vi "Lookup API by ID.vi"(8 "error in (no error)":errorcluster, 10 "API ID":string, 11 "VolatusCoreTask in":refnum<class "VolatusCoreTask.lvclass">) -> (0 "error out":errorcluster, 2 "API":refnum<class "API.lvclass">, 3 "VolatusCoreTask out":refnum<class "VolatusCoreTask.lvclass">)   [LabVIEW 2020, in "Volatus.lvlib" / "VolatusCoreTask.lvclass"]
uses:
  VolatusCoreTask.lvclass
  VolatusCoreTask.lvclass/VolatusCoreTask.ctl
  API/API.lvclass
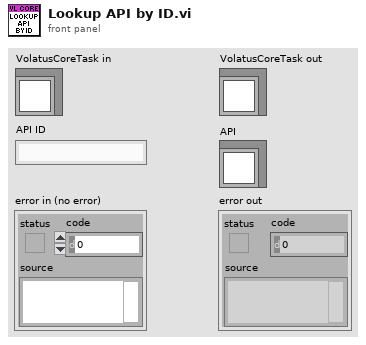
[diagram p1: front panel]
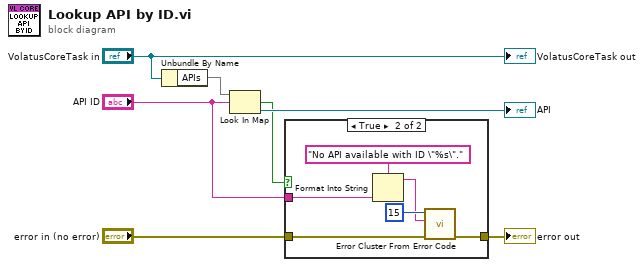
[diagram p0: block diagram]
diagram:
  n1 = Unbundle By Name("VolatusCoreTask in") -> ("APIs"=w6:map{string, refnum<class "API.lvclass">})
  n2 = Look In Map(map=w6, key="API ID") -> (key not found?=w4:bool, value=→"API":refnum<class "API.lvclass">)  [unwired: 1 in]
  n3 = case shown="True" w4 {
    tunnel: "API ID" -> [_ w13]
    tunnel: "error in (no error)" -> [w8 w10]
    tunnel: [w8 w9] -> w1
    frame False {
    }
    frame True {
      n4 = Format Into String(format string="No API available with ID \"%s\".", w13) -> (resulting string=w11:string)  [unwired: 2 in, 1 out]
      n5 = call <vilib>:"Error Cluster From Error Code.vi"("error in (no error)"=w10, "error message (\"\")"=w11, "error code (0)"=15) -> ("error out"=w9:errorcluster)  [unwired: 6 in]
    }
  }
  "error out" <- w1
  "VolatusCoreTask out" <- "VolatusCoreTask in"
